vi "Clock.vi"   [LabVIEW 2009]
doc: "I. Description:\nThis example demonstrates how to generate a continuous digital pulse train from a Counter Output Channel. The Frequency, Duty Cycle, and Idle State are all configurable. \n\nThis example shows how to configure the pulse in terms of Frequency/Duty Cycle, but can easily be modified to generate a pulse in terms of Time or Ticks.\n\nII. Instructions for Running:\n1. Select the Physical Channel which corresponds to the counter you want to output your signal to on the DAQ device.\n2. Enter the Frequency and Duty Cycle to define the pulse parameters. You can also change the Idle State to determine the beginning and end states of the output. If the Idle State is High, the generation will use inverted logic. Additionally, you can set the Initial Delay (in seconds) which will delay the beginning of the pulse train from the start call; this is currently wired to 0.0 on the diagram. \nNote: Use the Measure Period example to verify you are outputting the pulse train on the DAQ device.\n\nIII. Block Diagram Steps:\n1. Create a Counter Output channel to produce a Pulse in terms of Frequency. If the Idle State of the pulse is set to low, the state of the line will begin low and remain low after the generation is stopped.\n2. Use the DAQmx Timing VI (Implicit) to configure the duration of the pulse generation.\n3. Call the Start VI to arm the counter and begin the pulse train generation.\n4. Loop continuously until the user presses the Stop button. Check for errors every 100 ms using the Is Task Done? VI\n5. Call the Clear Task VI to clear the Task.\n\nIV. I/O Connections Overview:\nThe counter will output the pulse train on the output terminal of the counter specified in the Physical Channel I/O control. \n\nIn this example the output will be sent to the default output terminal on ctr0.\n\nFor more information on the default counter input and output terminals for your device, open the NI-DAQmx Help, and refer to Counter Signal Connections found under the Device Considerations book in the table of contents."
uses:
  <vilib>/DAQmx/configure/timing.llb/DAQmx Timing (Implicit).vi
  <vilib>/DAQmx/create/channels.llb/DAQmx Create Channel (CO-Pulse Generation-Frequency).vi
panel:
  # "For instructions, select Help>>Show Context Help"
  # "Channel Parameters"
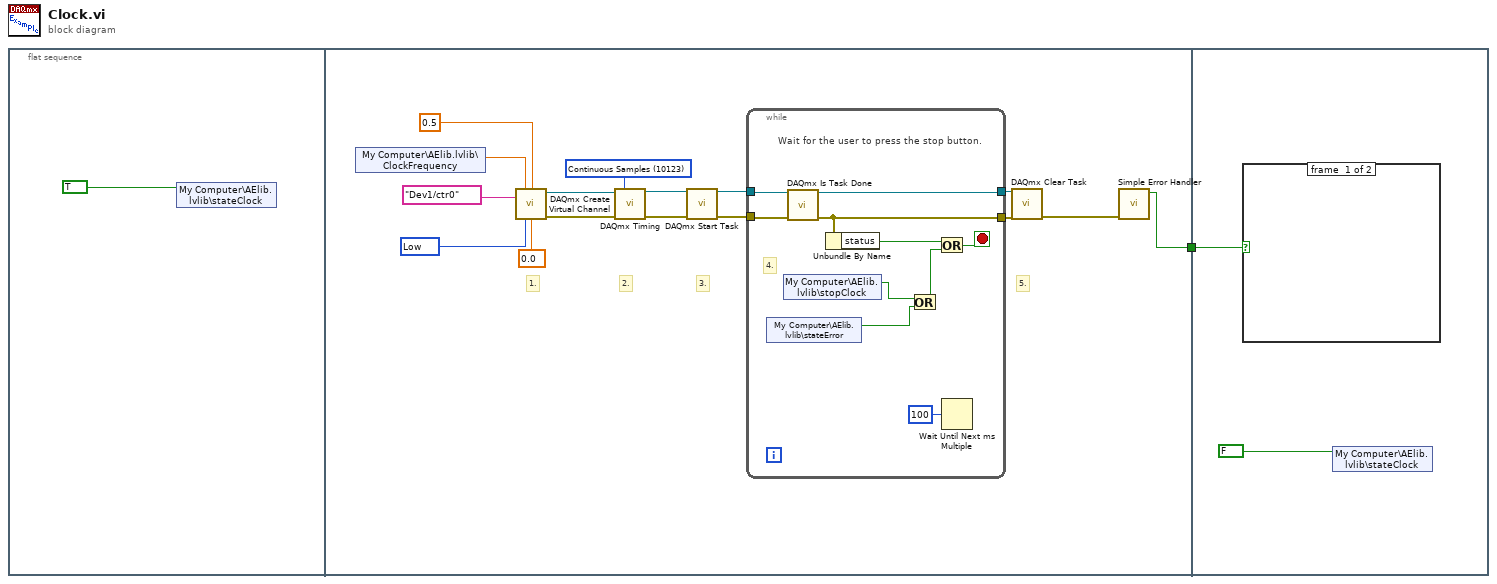
[diagram p0: block diagram]
diagram:
  n1 = flat-sequence {
    tunnel: [w4] -> w1
    tunnel: w1 -> [w30]
    frame #0 {
      n2 = shared-variable "My Computer\\AElib.lvlib\\stateClock"(TRUE) -> ()  [unwired: 1 in, 1 out]
    }
    frame #1 {
      w15 = 10214 items=["High"=10192, "Low"=10214] ("Idle State")
      w13 = 10123 items=["Finite Samples"=10178, "Continuous Samples"=10123] ("sample mode")
      # "5."
      # "3."
      # "2."
      # "1."
      n3 = shared-variable "My Computer\\AElib.lvlib\\ClockFrequency"() -> (w3:dbl)  [unwired: 1 in, 1 out]
      n4 = call-poly <vilib>:"DAQmx Create Virtual Channel.vi"("frequency"=w3, "duty cycle"=0.5 ("Duty Cycle"), "counter"=tag "Dev1/ctr0" ("Counter(s)"), "idle state"=w15, "initial delay"=0.0) -> ("task out"=w8:refnum<k21>, "error out"=w5:errorcluster)  [unwired: 9 in]
      n5 = call-poly <vilib>:"DAQmx Timing.vi"("task/channels in"=w8, "sample mode"=w13, "error in"=w5) -> ("task out"=w12:refnum<k21>, "error out"=w11:errorcluster)  [unwired: 11 in]
      n6 = call <vilib>:"DAQmx Start Task.vi"("task/channels in"=w12, "error in"=w11) -> ("task out"=w9:refnum<k21>, "error out"=w6:errorcluster)  [unwired: 12 in]
      n7 = while {
        tunnel: w6 -> [w27]
        tunnel: w9 -> [w28]
        tunnel: [w26] -> w10
        tunnel: [w25] -> w18
        stop <- w24 stop-if-true
        # "Wait for the user to press the stop button."
        # "4."
        n8 = shared-variable "My Computer\\AElib.lvlib\\stateError"() -> (w20:bool)  [unwired: 1 in, 1 out]
        n9 = shared-variable "My Computer\\AElib.lvlib\\stopClock"() -> (w19:bool)  [unwired: 1 in, 1 out]
        n10 = call <vilib>:"DAQmx Is Task Done.vi"("task/channels in"=w28, "error in"=w27) -> ("task out"=w26:refnum<k21>, "error out"=w25:errorcluster)  [unwired: 11 in, 1 out]
        n11 = Unbundle By Name(w25) -> ("status"=w22:bool)
        n12 = Or(x=w19, y=w20) -> (x .or. y?=w21:bool)
        n13 = Or(x=w22, y=w21) -> (x .or. y?=w24:bool)
        n14 = Wait Until Next ms Multiple(millisecond multiple=u32 100) -> ()  [unwired: 1 out]
      }
      n15 = call <vilib>:"DAQmx Clear Task.vi"("task in"=w10, "error in"=w18) -> ("error out"=w7:errorcluster)  [unwired: 13 in]
      n16 = call <vilib>:"Simple Error Handler.vi"("error in (no error)"=w7) -> ("error?"=w4:bool)  [unwired: 4 in, 4 out]
    }
    frame #2 {
      n17 = case shown="False" w30 {
        frame #0 {
        }
        frame #1 {
        }
      }
      n18 = shared-variable "My Computer\\AElib.lvlib\\stateClock"(FALSE) -> ()  [unwired: 1 in, 1 out]
    }
  }
